vi "process.vi"(8 "error in (no error)":errorcluster, 9 "Calling VI Reference i":refnum<vi>, 10 "Node Refnum":refnum<vi>, 11 "EventStructure in":refnum<class "EventStructure.lvclass">) -> (0 "error out":errorcluster, 3 "EventStructure out":refnum<class "EventStructure.lvclass">)   [LabVIEW 2016]
uses:
  Dependency/Dependency.lvclass
  Node/Node.lvclass
  EventStructure.lvclass
  C:/LSST_TS/SystemSW/ct_tools/Node/Node.lvclass
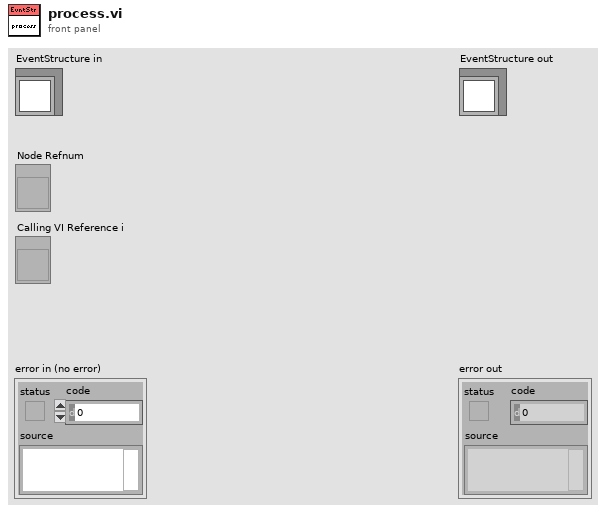
[diagram p1: front panel]
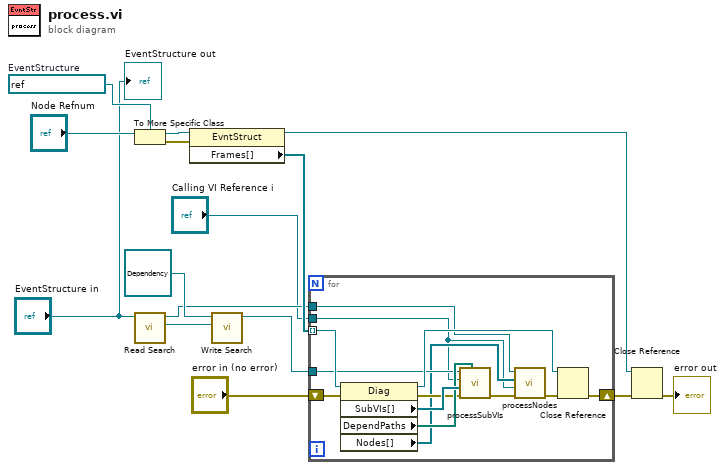
[diagram p0: block diagram]
diagram:
  w14 = refnum<vi> refnum  # EventStructure
  n1 = To More Specific Class(target class=w14, reference="Node Refnum") -> (specific class reference=w1:refnum<vi>, error out=w15:errorcluster)  [unwired: 1 in]
  n2 = call "Read Search.vi"("Node in"="EventStructure in") -> ("Search"=w10:refnum<class "Search.lvclass">, "Node out"=w6:refnum<class "EventStructure.lvclass">)  [unwired: 9 in]
  n3 = property class="EvntStruct"(reference=w1, error in=w15) -> (reference out=w12:refnum<vi>, "Frames[]"=w8:refnum<vi>[])  [unwired: 1 out]
  n4 = call "Write Search.vi"("Search"=w10, "Dependency in"=refnum<class "Dependency.lvclass"> refnum ("Dependency.lvclass")) -> ("Dependency out"=w2:refnum<class "Dependency.lvclass">)  [unwired: 9 in]
  n5 = for {
    tunnel: w8 -> [w28] mode=indexing
    tunnel: "Calling VI Reference i" -> [w16]
    shift-right: [w22] -> w13
    shift-left: "error in (no error)" -> [w25]
    tunnel: w2 -> [w21]
    tunnel: w6 -> [w20]
    n6 = property class="Diag"(reference=w28, error in=w25) -> (reference out=w23:refnum<vi>, error out=w24:errorcluster, "SubVIs[]"=w27:refnum<vi>[], "DependPaths"=w26:path[], "Nodes[]"=w19:refnum<vi>[])
    n7 = call "processSubVIs.vi"("VIDependencyPaths"=w26, "error in (no error)"=w24, "SubVIs[]"=w27, "Calling VI Reference i"=w16, "Dependency in"=w21) -> ("error out"=w18:errorcluster)  [unwired: 4 in, 2 out]
    n8 = call "processNodes.vi"("error in (no error)"=w18, "Calling VI Reference i"=w16, "Nodes[]"=w19, "Node in"=w20) -> ("error out"=w17:errorcluster)  [unwired: 6 in, 1 out]
    n9 = Close Reference(reference=w23, error in (no error)=w17) -> (error out=w22:errorcluster)
  }
  n10 = Close Reference(reference=w12, error in (no error)=w13) -> (error out=→"error out":errorcluster)
  "EventStructure out" <- "EventStructure in"
